vi "Function.vi"(8 "error in (no error)":errorcluster, 9 "B":T1, 10 "A":T1, 11 "OR in":refnum<class "OR_I8.lvclass">) -> (0 "error out":errorcluster, 2 "Result":T1, 3 "OR out":refnum<class "OR_I8.lvclass">)   [LabVIEW 2021, in "OR_I8.lvclass"]
uses:
  OR_I8.lvclass
  Type.ctl
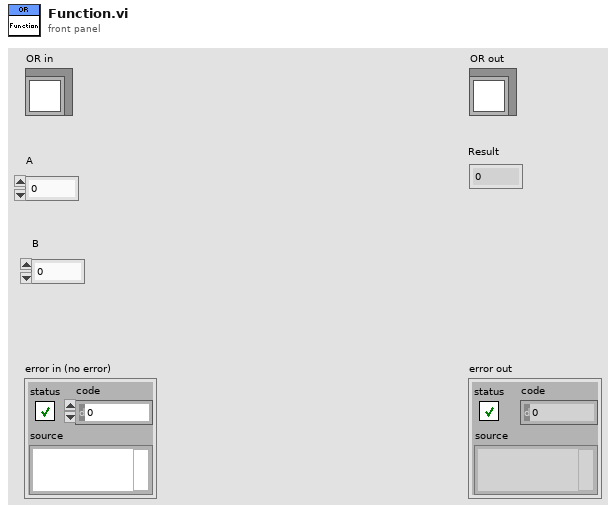
[diagram p1: front panel]
types:
  T1 = typedef "OR_I8.lvclass/Type.ctl" = i8
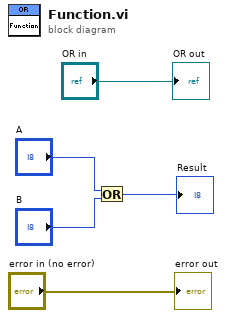
[diagram p0: block diagram]
diagram:
  n1 = Or(x="A", y="B") -> (x .or. y?=→"Result":T1)
  "error out" <- "error in (no error)"
  "OR out" <- "OR in"
